vi "ChooseTarget.vi"(4 "WayPointProb":dbl format="%#_13g", 6 "GoalProb":dbl format="%#_13g", 8 "Field Geometry":dbl[](array[numeric])=[0.0, 999999.0, 999999.0, -1.0], 9 "WayPointCache":dbl[][](array[numeric]), 10 "Goal":dbl[](array[numeric])) -> (2 "Target":dbl[](array[numeric]))   [LabVIEW 2017]
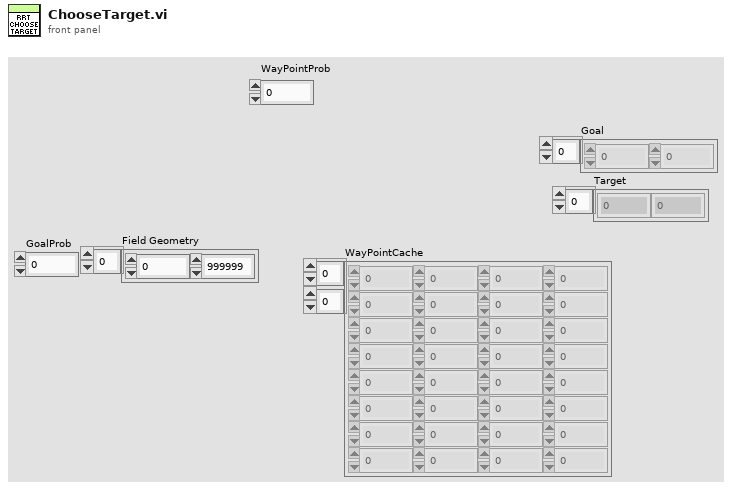
[diagram p1: front panel]
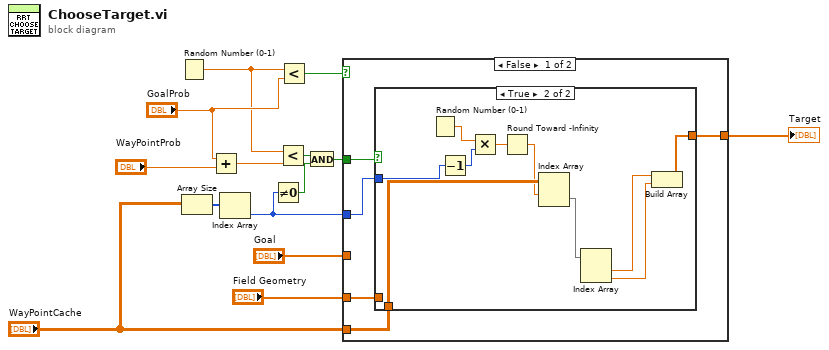
[diagram p0: block diagram]
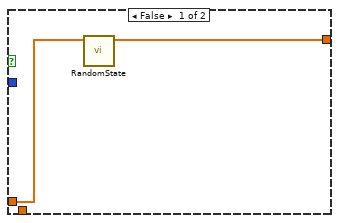
[diagram p2: hidden frame]
diagram:
  n1 = Random Number (0-1)() -> (number: 0 to 1=w7:dbl)
  n2 = Array Size(array="WayPointCache") -> (size(s)=w4:i32[])
  n3 = Add(x="GoalProb", y="WayPointProb") -> (x+y=w10:dbl)
  n4 = Index Array(array=w4) -> (element=w1:i32)  [unwired: 1 in]
  n5 = Not Equal To 0?(x=w1) -> (x != 0?=w2:bool)
  n6 = Less?(x=w7, y=w10) -> (x < y?=w6:bool)
  n7 = Less?(x=w7, y="GoalProb") -> (x < y?=w14:bool)
  n8 = And(x=w6, y=w2) -> (x .and. y?=w5:bool)
  n9 = case shown="False" w14 {
    tunnel: "Goal" -> [_ w32]
    tunnel: [w19 w32] -> w11
    tunnel: "Field Geometry" -> [w18 _]
    tunnel: w5 -> [w17 _]
    tunnel: "WayPointCache" -> [w16 _]
    tunnel: w1 -> [w15 _]
    frame False {
      n10 = case shown="True" w17 {
        tunnel: [w21 w24] -> w19
        tunnel: w18 -> [w20 _]
        tunnel: w16 -> [_ w29]
        tunnel: w15 -> [_ w23]
        frame False {
          n11 = call "RandomState.vi"("Field Geometry"=w20) -> ("Array"=w21:dbl[])  [unwired: 10 in]
        }
        frame True {
          n12 = Random Number (0-1)() -> (number: 0 to 1=w31:dbl)
          n13 = Decrement(x=w23) -> (x-1=w22:i32)
          n14 = Multiply(x=w31, y=w22) -> (x*y=w30:dbl)
          n15 = Round Toward -Infinity(1:w30) -> (0:w28:dbl)
          n16 = Index Array(array=w29, index (row)=w28) -> (element=w27:dbl[])  [unwired: 1 in]
          n17 = Index Array(array=w27) -> (element #1=w26:dbl, element #2=w25:dbl)  [unwired: 2 in]
          n18 = Build Array(w26, w25) -> (w24:dbl[])
        }
      }
    }
    frame True {
    }
  }
  "Target" <- w11
